vi "2022_day5_sub_parser.vi"(11 "Data":T1) -> (0 "Crane Stock (for Algorithm)":string[](array[string]), 3 "Rearrangement Procedure":cluster{"move":i32, "from":i32, "to":i32}[](array[cluster]), 7 "Crane Stock (Table)":string[][](array[string]))   [LabVIEW 2021]
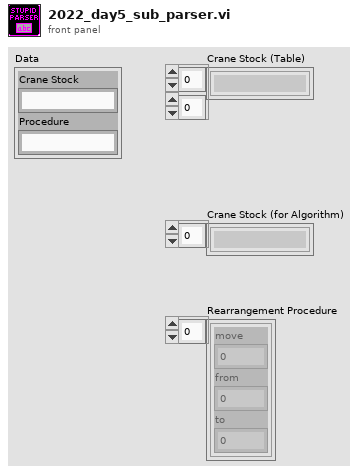
[diagram p1: front panel]
types:
  T1 = cluster{"Crane Stock":string, "Procedure":string}
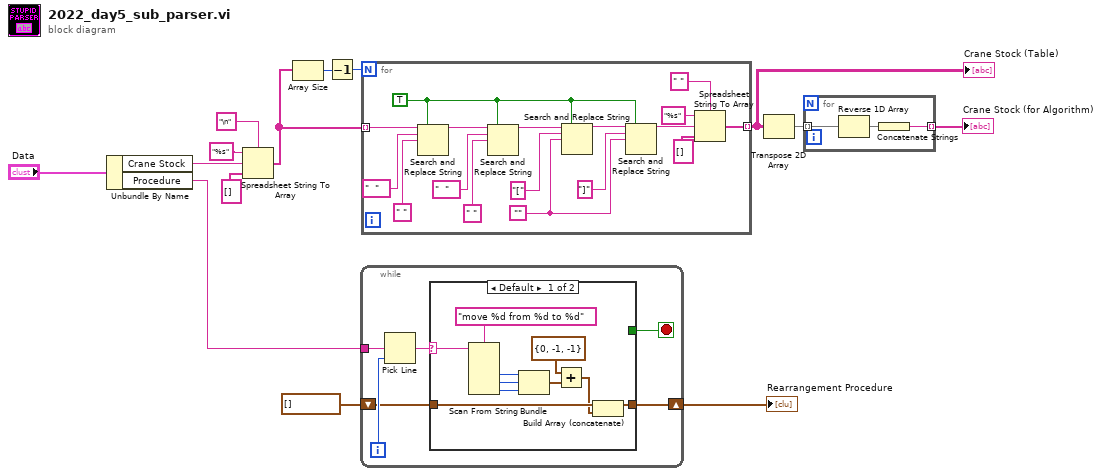
[diagram p0: block diagram]
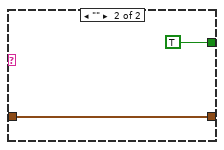
[diagram p2: hidden frame]
diagram:
  n1 = Unbundle By Name("Data") -> ("Crane Stock"=w8:string, "Procedure"=w9:string)
  n2 = Spreadsheet String To Array(delimiter (Tab)="\n", format string="%s", spreadsheet string=w8, array type (2D Dbl)=string[] []) -> (array=w4:string[])
  n3 = Array Size(array=w4) -> (size(s)=w5:i32)
  n4 = Decrement(x=w5) -> (x-1=w6:i32)
  n5 = while {
    tunnel: w9 -> [w20]
    shift-right: [w16] -> w14
    shift-left: cluster{"move":i32, "from":i32, "to":i32}[] [] -> [w15]
    i -> [w19]
    stop <- w17 stop-if-true
    n6 = Pick Line(multi-line string=w20, line index=w19) -> (output string=w18:string)  [unwired: 1 in]
    n7 = case shown="Default" w18 {
      selector: w18 -> [w30 _]
      tunnel: [_ TRUE] -> w17
      tunnel: [w25 w31] -> w16
      tunnel: w15 -> [w24 w31]
      frame Default {
        n8 = Scan From String(format string="move %d from %d to %d", input string=w30) -> (output 1=w28:i32, output 2=w27:i32, output 3=w26:i32)  [unwired: 5 in, 3 out]
        n9 = Bundle(w28, w27, w26) -> (w23:cluster{i32, i32, i32})  [unwired: 1 in]
        n10 = Add(x=cluster{"move":i32, "from":i32, "to":i32} {"move"=0, "from"=-1, "to"=-1}, y=w23) -> (x+y=w22:cluster{i32, i32, i32})
        n11 = Build Array (concatenate)(w24, w22) -> (w25:cluster{"move":i32, "from":i32, "to":i32}[])
      }
      frame "" {
      }
    }
  }
  "Rearrangement Procedure" <- w14
  n12 = for {
    N: w6 -> [_]
    tunnel: w4 -> [w40] mode=indexing
    tunnel: [w46] -> w12 mode=indexing
    w33 = TRUE ("replace all? (F)")
    w41 = ""
    n13 = Search and Replace String(replace all?=w33, input string=w40, search string="  " ("delimiter (Tab)"), replace string=" " ("delimiter (Tab)")) -> (result string=w35:string)  [unwired: 4 in, 3 out]
    n14 = Search and Replace String(replace all?=w33, input string=w35, search string="  " ("delimiter (Tab)"), replace string=" " ("delimiter (Tab)")) -> (result string=w34:string)  [unwired: 4 in, 3 out]
    n15 = Search and Replace String(replace all?=w33, input string=w34, search string="[" ("input string"), replace string=w41) -> (result string=w45:string)  [unwired: 4 in, 3 out]
    n16 = Search and Replace String(replace all?=w33, input string=w45, search string="]", replace string=w41) -> (result string=w42:string)  [unwired: 4 in, 3 out]
    n17 = Spreadsheet String To Array(delimiter (Tab)=" ", format string="%s", spreadsheet string=w42, array type (2D Dbl)=string[] []) -> (array=w46:string[])
  }
  "Crane Stock (Table)" <- w12
  n18 = Transpose 2D Array(2D array=w12) -> (transposed array=w11:string[][])
  n19 = for {
    tunnel: w11 -> [w52] mode=indexing
    tunnel: [w51] -> w13 mode=indexing
    n20 = Reverse 1D Array(array=w52) -> (reversed array=w50:string[])
    n21 = Concatenate Strings(w50) -> (w51:string)
  }
  "Crane Stock (for Algorithm)" <- w13
